vi "ROSServiceRead.vi"(0 "error in":errorcluster, 1 "vi reference":refnum<vi>) -> (2 "error out":errorcluster, 3 "Reply":string, 4 "vi reference":refnum<vi>)   [LabVIEW 2012]
doc: "Attempts to wait for a response from a server call before returning an empty string. Implemented in ROS_Topic_Read."
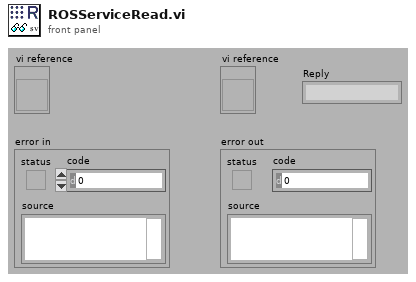
[diagram p1: front panel]
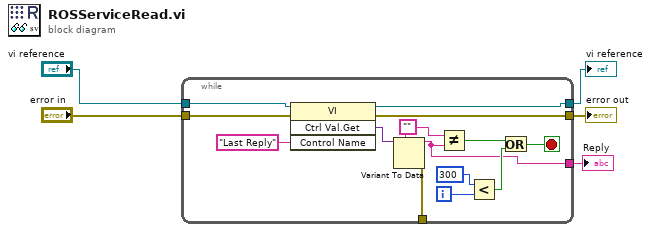
[diagram p0: block diagram]
diagram:
  n1 = while {
    tunnel: "vi reference" -> [w19]
    tunnel: [w18] -> w4
    tunnel: [w17] -> w5
    tunnel: "error in" -> [w16]
    tunnel: [w7] -> w3
    tunnel: [w6] -> _
    i -> [w13]
    stop <- w10 stop-if-true
    w9 = ""
    n2 = invoke class="VI" method="Ctrl Val.Get"(reference=w19, error in=w16, "Control Name"="Last Reply") -> (reference out=w18:refnum<vi>, error out=w17:errorcluster, "Get Control Value Variant"=w14:variant)  [unwired: 1 in, 1 out]
    n3 = Variant To Data(type=w9, Variant=w14) -> (data=w7:string, error out=w6:errorcluster)  [unwired: 1 in]
    n4 = Not Equal?(x=w9, y=w7) -> (x != y?=w8:bool)
    n5 = Less?(x=300, y=w13) -> (x < y?=w11:bool)
    n6 = Or(x=w8, y=w11) -> (x .or. y?=w10:bool)
  }
  "error out" <- w5
  "vi reference" <- w4
  "Reply" <- w3
